vi "Asynchronous Logging Loop.vi"(8 "error in (no error)":errorcluster, 11 "Log Data FIFO":refnum<k33>) -> (0 "error out":errorcluster)   [LabVIEW 2019, in "Inline Telemetry Prototype Engine.lvlib"]
uses:
  Inline Telemetry Prototype Engine.lvlib
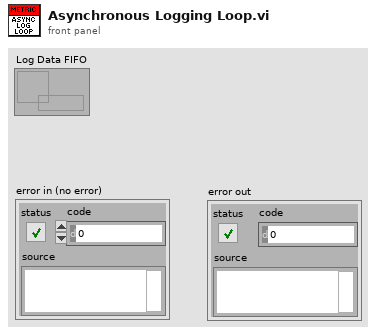
[diagram p1: front panel]
types:
  T1 = enum16{"open", "open or create", "create or replace", "create", "open (read-only)"}
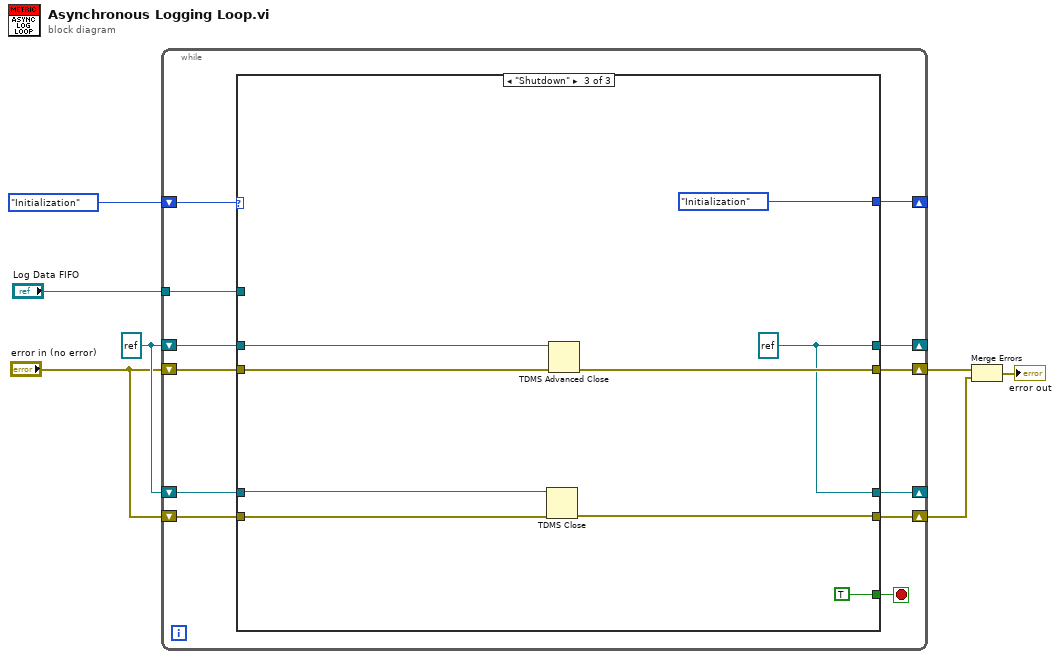
[diagram p0: block diagram]
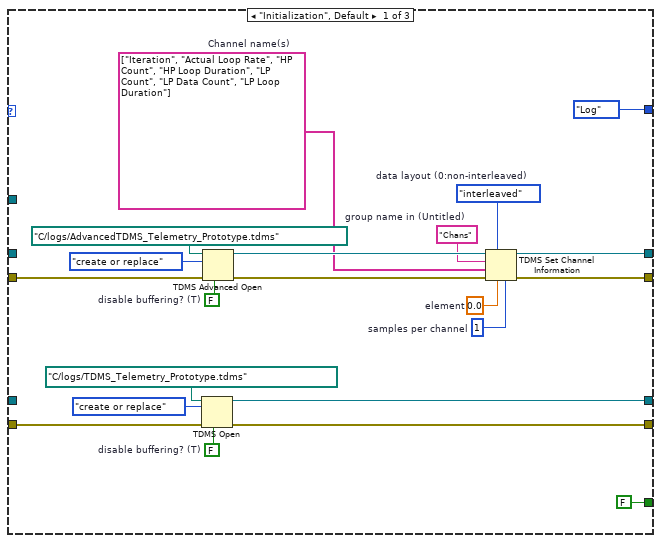
[diagram p2: hidden frame]
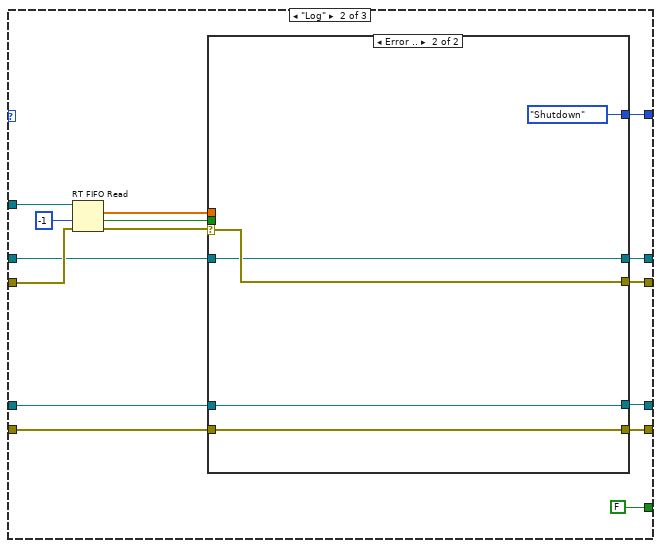
[diagram p3: hidden frame]
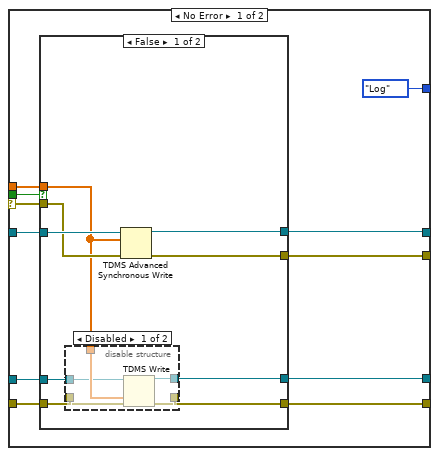
[diagram p4: hidden frame]
diagram:
  w4 = refnum<k34> refnum ("tdms file out")
  n1 = while {
    shift-right: [w17] -> _
    shift-left: enum16{"Initialization", "Log", "Shutdown"}."Initialization" -> [w18]
    shift-right: [w16] -> w5
    shift-left: "error in (no error)" -> [w19]
    shift-right: [w14] -> _
    shift-left: w4 -> [w13]
    tunnel: "Log Data FIFO" -> [w12]
    shift-right: [w11] -> _
    shift-left: w4 -> [w10]
    shift-right: [w8] -> w1
    shift-left: "error in (no error)" -> [w9]
    stop <- w15 stop-if-true
    n2 = case shown="\"Shutdown\"" w18 {
      tunnel: w19 -> [w27 w51 w97]
      tunnel: [enum16{"Initialization", "Log", "Shutdown"}."Log" w55 enum16{"Initialization", "Log", "Shutdown"}."Initialization"] -> w17
      tunnel: [w30 w46 w96] -> w16
      tunnel: [FALSE FALSE TRUE] -> w15
      tunnel: [w29 w45 w90] -> w14
      tunnel: w13 -> [_ w47 w95]
      tunnel: w12 -> [_ w53 _]
      tunnel: [w22 w41 w90] -> w11
      tunnel: w10 -> [_ w42 w92]
      tunnel: [w21 w43 w91] -> w8
      tunnel: w9 -> [w20 w44 w93]
      frame "Initialization", Default {
        w23 = FALSE  # disable buffering? (T)
        w34 = enum16{"non-interleaved", "interleaved"}."interleaved"  # data layout (0:non-interleaved)
        w36 = u32 1  # samples per channel
        w35 = 0.0  # element
        w32 = "Chans"  # group name in (Untitled)
        w38 = FALSE  # disable buffering? (T)
        w33 = string[] ["Iteration", "Actual Loop Rate", "HP Count", "HP Loop Duration", "LP Count", "LP Data Count", "LP Loop Duration"]  # Channel name(s)
        n3 = TDMS Open(6:w23, 8:w20, 10:T1."create or replace" ("operation (0:open)"), 11:path "C:/logs/TDMS_Telemetry_Prototype.tdms" ("file path")) -> (0:w21:errorcluster, 3:w22:refnum<k34>)  [unwired: 3 in]
        n4 = TDMS Advanced Open(6:w38, 8:w27, 10:T1."create or replace" ("operation (0:open)"), 11:path "C:/logs/AdvancedTDMS_Telemetry_Prototype.tdms" ("file path")) -> (0:w39:errorcluster, 3:w40:refnum<k34>)  [unwired: 1 in, 1 out]
        n5 = TDMS Set Channel Information(4:w36, 6:w35, 7:w34, 8:w39, 9:w33, 10:w32, 11:w40) -> (0:w30:errorcluster, 3:w29:refnum<k34>)
      }
      frame "Log" {
        n6 = RT FIFO Read(0:w53, 2:-1 ("timeout in ms (0)"), 3:w51) -> (9:w49:dbl[], 10:w48:bool, 11:w50:errorcluster)  [unwired: 1 in, 2 out]
        n7 = case shown="Error .." w50 {
          selector: w50 -> [w63 w88]
          tunnel: [enum16{"Initialization", "Log", "Shutdown"}."Log" enum16{"Initialization", "Log", "Shutdown"}."Shutdown"] -> w55
          tunnel: w49 -> [w60 _]
          tunnel: w48 -> [w65 _]
          tunnel: w47 -> [w64 w87]
          tunnel: [w62 w88] -> w46
          tunnel: [w61 w87] -> w45
          tunnel: w44 -> [w59 w85]
          tunnel: [w58 w85] -> w43
          tunnel: w42 -> [w57 w86]
          tunnel: [w56 w86] -> w41
          frame No Error {
            n8 = case shown="False" w65 {
              tunnel: w64 -> [w75 w83]
              tunnel: w63 -> [w74 w84]
              tunnel: [w73 w84] -> w62
              tunnel: [w72 w83] -> w61
              tunnel: w60 -> [w67 _]
              tunnel: w59 -> [w71 w81]
              tunnel: [w70 w81] -> w58
              tunnel: w57 -> [w69 w82]
              tunnel: [w68 w82] -> w56
              frame False {
                n9 = disable-structure shown="Disabled" {
                  disable-tunnel: w71 -> [w80 _]
                  disable-tunnel: w67 -> [w79 _]
                  disable-tunnel: [w78 _] -> w70
                  disable-tunnel: w69 -> [w77 _]
                  disable-tunnel: [w76 _] -> w68
                  frame Disabled {
                    n10 = TDMS Write(0:w77, 9:w79, 11:w80) -> (4:w76:refnum<k34>, 15:w78:errorcluster)  [unwired: 3 in, 2 out]
                  }
                  frame Enabled {
                  }
                }
                n11 = TDMS Advanced Synchronous Write(8:w74, 10:w67, 11:w75) -> (0:w73:errorcluster, 3:w72:refnum<k34>)
              }
              frame True {
              }
            }
          }
          frame Error {
          }
        }
      }
      frame "Shutdown" {
        w90 = refnum<k34> refnum ("tdms file out")
        n12 = TDMS Close(8:w93, 11:w92) -> (0:w91:errorcluster)  [unwired: 1 out]
        n13 = TDMS Advanced Close(8:w97, 11:w95) -> (0:w96:errorcluster)  [unwired: 2 in, 1 out]
      }
    }
  }
  n14 = Merge Errors(w5, w1) -> (→"error out":errorcluster)
